vi "ChipKit Blink (Digital Write).vi"() -> ()   [LabVIEW 2011, in "LabVIEW Interface for ChipKit.lvlib"]
uses:
  vi.lib/LabVIEW Interface for ChipKit/LabVIEW Interface for ChipKit.lvlib
  vi.lib/LabVIEW Interface for ChipKit/Private/Type Defs/Chipkit Resource.ctl
  vi.lib/LabVIEW Interface for ChipKit/Private/Type Defs/Board Type.ctl
  vi.lib/LabVIEW Interface for ChipKit/Private/Type Defs/Connection Type.ctl
  vi.lib/LabVIEW Interface for ChipKit/Private/Type Defs/Pin Mode.ctl
panel:
  out "User LED":bool
  in  "Blink Period (ms)":u32=1000
  in  "ChipKit Configuration":T1={"COM Port"="COM3", "Board Type"=enum."ChipKit uC32", "Connection Type"=enum."USB / Serial", "Baud Rate (115200)"=115200, "Bytes Per Packet (15)"=15}
  in  "Stop Button":bool
  # "Blink Example\n\nThis example demonstrates how to blink the user LED on the ChipKit at various frequencies.\n\nInstructions\n1. Select the COM Port associated with the ChipKit.\n2. Select the Board Type.\n3. Click the Run Arrow.\n4. Adjust the Blink Period to change the blink rate of the LED."
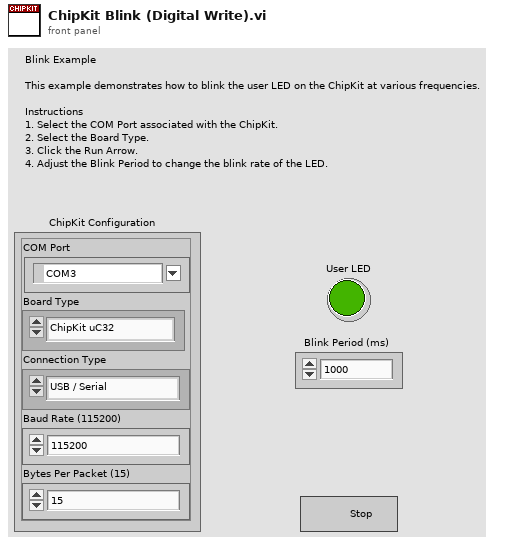
[diagram p1: front panel]
types:
  T1 = typedef "LabVIEW Interface for ChipKit.lvlib/Chipkit Resource.ctl" = cluster{"COM Port":refnum<visa-resource-name>, "Board Type":T2, "Connection Type":T3, "Baud Rate (115200)":u32, "Bytes Per Packet (15)":u32}
  T2 = typedef "LabVIEW Interface for ChipKit.lvlib/Board Type.ctl" = enum16{"ChipKit uC32", "ChipKit Uno32", "ChipKit Max32"}
  T3 = typedef "LabVIEW Interface for ChipKit.lvlib/Connection Type.ctl" = enum8{"USB / Serial", "XBEE", "BlueSmirf (Bluetooth)"}
  T4 = typedef "LabVIEW Interface for ChipKit.lvlib/Pin Mode.ctl" = enum16{"Input", "Output"}
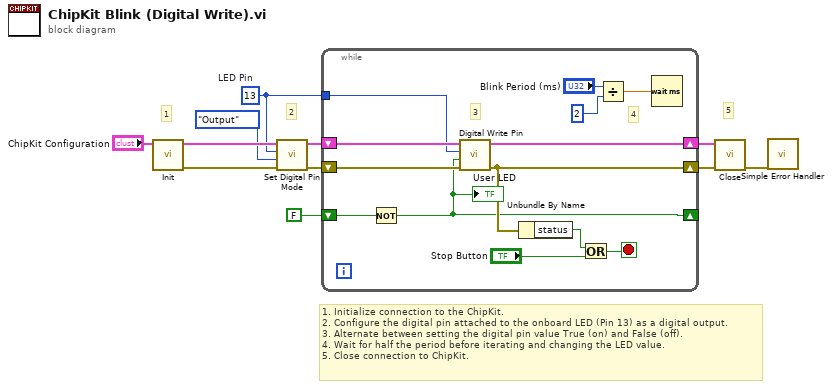
[diagram p0: block diagram]
diagram:
  w1 = u8 13  # LED Pin
  # "2"
  # "1. Initialize connection to the ChipKit.\n2. Configure the digital pin attached to the onboard LED (Pin 13) as a digital output.\n3. Alternate between setting the digital pin value True (on) and False (off).\n4. Wait for half the period before iterating and changing the LED value. \n5. Close connection to ChipKit."
  # "5"
  # "1"
  n1 = call "Init.vi"("ChipKit Configuration"="ChipKit Configuration") -> ("Error Out"=w9:errorcluster, "ChipKit Configuration"=w4:T1)  [unwired: 9 in]
  n2 = call "Set Digital Pin Mode.vi"("Error In"=w9, "Pin Mode (Input)"=Pin_Mode."Output", "Digital I/O Pin"=w1, "Arduino Resource"=w4) -> ("Error Out"=w5:errorcluster, "Arduino Resource"=w3:T1)  [unwired: 6 in]
  n3 = while {
    shift-right: [w24] -> w11
    shift-left: w3 -> [w20]
    shift-right: [w23] -> w10
    shift-left: w5 -> [w19]
    shift-right: [w16] -> _
    shift-left: FALSE -> [w17]
    tunnel: w1 -> [w12]
    stop <- w22 stop-if-true
    # "4"
    # "3"
    n4 = Not(x=w17) -> (.not. x?=w16:bool)
    "User LED" <- w16
    n5 = call "Digital Write Pin.vi"("Error In"=w19, "Value (Off)"=w16, "Digital I/O Pin (2)"=w12, "ChipKit Resource"=w20) -> ("Error Out"=w23:errorcluster, "ChipKit Resource"=w24:T1)  [unwired: 6 in]
    n6 = Unbundle By Name(w23) -> ("status"=w21:bool)
    n7 = Or(x=w21, y="Stop Button") -> (x .or. y?=w22:bool)
    n8 = Divide(x="Blink Period (ms)", y=u32 2) -> (x/y=w13:dbl)
    n9 = Wait (ms)(milliseconds to wait=w13) -> ()  [unwired: 1 out]
  }
  n10 = call "Close.vi"("Error In"=w10, "ChipKit Configuration"=w11) -> ("Error Out"=w8:errorcluster)  [unwired: 9 in]
  n11 = call <vilib>:"Simple Error Handler.vi"("error in (no error)"=w8) -> ()  [unwired: 4 in, 5 out]
